vi "Generate Scan Settings File Name.vi"(7 "Setting File Type":T1=enum."Configuration Settings", 8 "error in (no error)":errorcluster, 11 "Settings Folder Path IN":path) -> (0 "error out":errorcluster, 2 "New Settings Filename":string, 3 "Settings File Path":path)   [LabVIEW 2012]
doc: "SciScan 1.2 160622"
uses:
  Custom Controls/Setting File Types.ctl
  <vilib>/regexp/Match Regular Expression.xnode
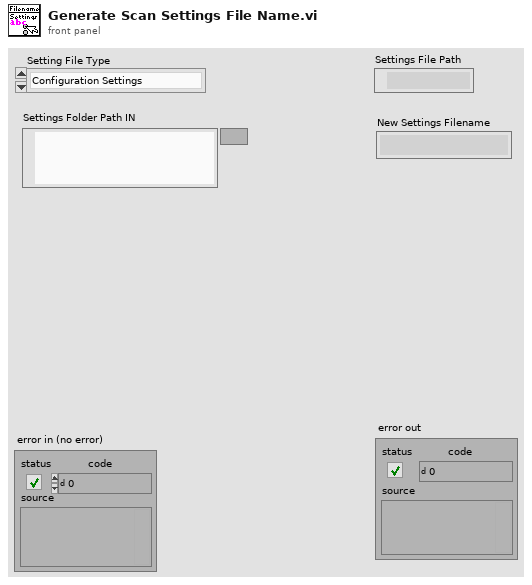
[diagram p1: front panel]
types:
  T1 = typedef "Setting File Types.ctl" = enum16{"2D.Frame.Scan.Settings", "2D.Line.Scan.Settings", "Z.Stack.Settings", "HW Settings", "Configuration Settings", "Unknown Settings", "Fast.Z.Settings"}
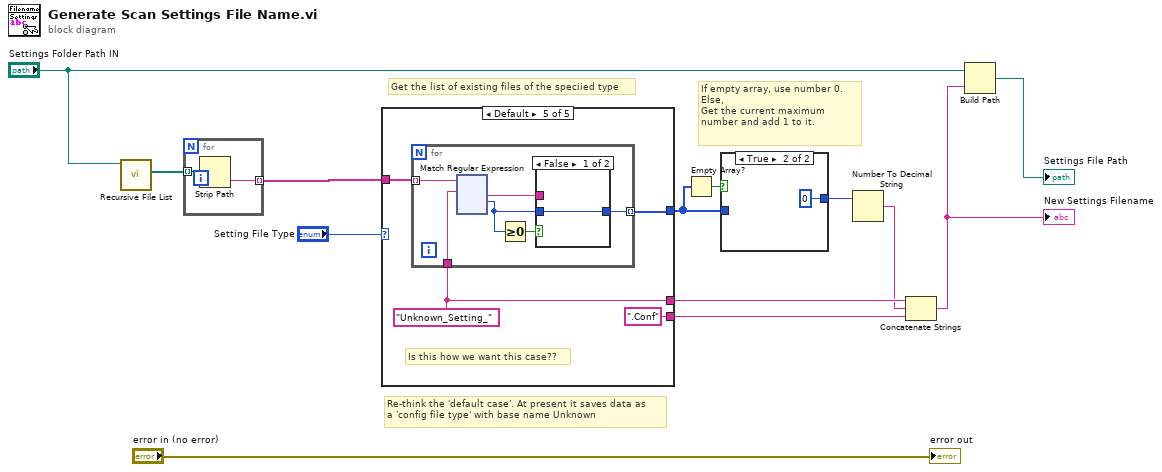
[diagram p0: block diagram]
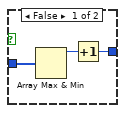
[diagram p2: hidden frame]
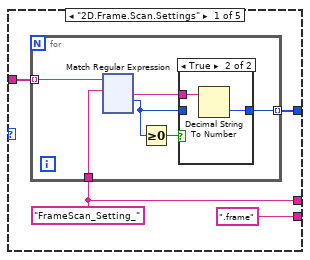
[diagram p3: hidden frame]
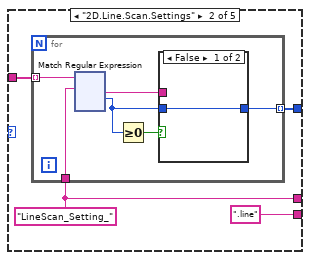
[diagram p5: hidden frame]
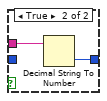
[diagram p6: hidden frame]
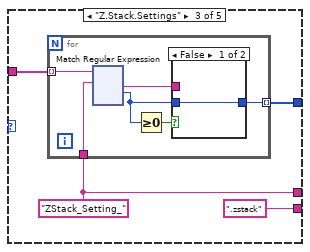
[diagram p7: hidden frame]
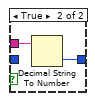
[diagram p8: hidden frame]
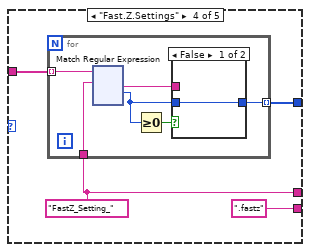
[diagram p9: hidden frame]
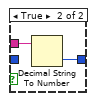
[diagram p10: hidden frame]
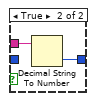
[diagram p11: hidden frame]
diagram:
  # "Re-think the 'default case'. At present it saves data as\na 'config file type' with base name Unknown"
  # "If empty array, use number 0.\nElse, \nGet the current maximum number and add 1 to it."
  # "Get the list of existing files of the speciied type"
  n1 = call <vilib>:"Recursive File List.vi"("Folder Path"="Settings Folder Path IN") -> ("All Files in Dir"=w8:path[])  [unwired: 6 in, 4 out]
  n2 = for {
    tunnel: w8 -> [w15] mode=indexing
    tunnel: [w14] -> w7 mode=indexing
    n3 = Strip Path(path=w15) -> (name=w14:string)  [unwired: 1 out]
  }
  n4 = case shown="Default" "Setting File Type" {
    tunnel: w7 -> [w19 w143 w267 w391 w513]
    tunnel: [w18 w142 w266 w390 w512] -> w6
    tunnel: [w16 w140 w264 w388 w514] -> w11
    tunnel: [".frame" ("Settings File Name IN") ".line" ("Settings File Name IN") ".zstack" ("Settings File Name IN") ".fastz" ("Settings File Name IN") ".Conf" ("Settings File Name IN")] -> w9
    frame "2D.Frame.Scan.Settings" {
      w16 = "FrameScan_Setting_" ("Settings File Name IN")
      n5 = for {
        tunnel: w19 -> [w24] mode=indexing
        tunnel: [w23] -> w18 mode=indexing
        tunnel: w16 -> [w22]
        n6 = xnode "Match Regular Expression"("input string"=w24, "regular expression"=w22) -> ("after match"=w25:string, "offset past match"=w20:i32)  [unwired: 4 in, 3 out]
        n7 = Greater Or Equal To 0?(x=w20) -> (x >= 0?=w21:bool)
        n8 = case shown="True" w21 {
          tunnel: w25 -> [_ w28]
          tunnel: [w26 w27] -> w23
          tunnel: w20 -> [w26 _]
          frame False {
          }
          frame True {
            n9 = Decimal String To Number(string=w28) -> (number=w27:i32)  [unwired: 2 in, 1 out]
          }
        }
      }
    }
    frame "2D.Line.Scan.Settings" {
      w140 = "LineScan_Setting_" ("Settings File Name IN")
      n10 = for {
        tunnel: w143 -> [w148] mode=indexing
        tunnel: [w147] -> w142 mode=indexing
        tunnel: w140 -> [w146]
        n11 = xnode "Match Regular Expression"("input string"=w148, "regular expression"=w146) -> ("after match"=w149:string, "offset past match"=w144:i32)  [unwired: 4 in, 3 out]
        n12 = Greater Or Equal To 0?(x=w144) -> (x >= 0?=w145:bool)
        n13 = case shown="False" w145 {
          tunnel: w149 -> [_ w152]
          tunnel: [w150 w151] -> w147
          tunnel: w144 -> [w150 _]
          frame False {
          }
          frame True {
            n14 = Decimal String To Number(string=w152) -> (number=w151:i32)  [unwired: 2 in, 1 out]
          }
        }
      }
    }
    frame "Z.Stack.Settings" {
      w264 = "ZStack_Setting_" ("Settings File Name IN")
      n15 = for {
        tunnel: w267 -> [w272] mode=indexing
        tunnel: [w271] -> w266 mode=indexing
        tunnel: w264 -> [w270]
        n16 = xnode "Match Regular Expression"("input string"=w272, "regular expression"=w270) -> ("after match"=w273:string, "offset past match"=w268:i32)  [unwired: 4 in, 3 out]
        n17 = Greater Or Equal To 0?(x=w268) -> (x >= 0?=w269:bool)
        n18 = case shown="False" w269 {
          tunnel: w273 -> [_ w276]
          tunnel: [w274 w275] -> w271
          tunnel: w268 -> [w274 _]
          frame False {
          }
          frame True {
            n19 = Decimal String To Number(string=w276) -> (number=w275:i32)  [unwired: 2 in, 1 out]
          }
        }
      }
    }
    frame "Fast.Z.Settings" {
      w388 = "FastZ_Setting_" ("Settings File Name IN")
      n20 = for {
        tunnel: w391 -> [w396] mode=indexing
        tunnel: [w395] -> w390 mode=indexing
        tunnel: w388 -> [w394]
        n21 = xnode "Match Regular Expression"("input string"=w396, "regular expression"=w394) -> ("after match"=w397:string, "offset past match"=w392:i32)  [unwired: 4 in, 3 out]
        n22 = Greater Or Equal To 0?(x=w392) -> (x >= 0?=w393:bool)
        n23 = case shown="False" w393 {
          tunnel: w397 -> [_ w400]
          tunnel: [w398 w399] -> w395
          tunnel: w392 -> [w398 _]
          frame False {
          }
          frame True {
            n24 = Decimal String To Number(string=w400) -> (number=w399:i32)  [unwired: 2 in, 1 out]
          }
        }
      }
    }
    frame Default {
      w514 = "Unknown_Setting_" ("Settings File Name IN")
      # "Is this how we want this case??"
      n25 = for {
        tunnel: w513 -> [w520] mode=indexing
        tunnel: [w519] -> w512 mode=indexing
        tunnel: w514 -> [w518]
        n26 = xnode "Match Regular Expression"("input string"=w520, "regular expression"=w518) -> ("after match"=w521:string, "offset past match"=w516:i32)  [unwired: 4 in, 3 out]
        n27 = Greater Or Equal To 0?(x=w516) -> (x >= 0?=w517:bool)
        n28 = case shown="False" w517 {
          tunnel: w521 -> [_ w524]
          tunnel: [w522 w523] -> w519
          tunnel: w516 -> [w522 _]
          frame False {
          }
          frame True {
            n29 = Decimal String To Number(string=w524) -> (number=w523:i32)  [unwired: 2 in, 1 out]
          }
        }
      }
    }
  }
  n30 = Empty Array?(array=w6) -> (empty?=w5:bool)
  n31 = case shown="True" w5 {
    tunnel: w6 -> [w638 _]
    tunnel: [w637 0] -> w12
    frame False {
      n32 = Array Max & Min(array=w638) -> (max value=w636:i32)  [unwired: 3 out]
      n33 = Increment(x=w636) -> (x+1=w637:i32)
    }
    frame True {
    }
  }
  n34 = Number To Decimal String(number=w12) -> (decimal integer string=w10:string)  [unwired: 1 in]
  n35 = Concatenate Strings(w11, w10, w9) -> (w2:string)
  "New Settings Filename" <- w2
  n36 = Build Path(base path="Settings Folder Path IN", name or relative path=w2) -> (appended path=→"Settings File Path":path)
  "error out" <- "error in (no error)"
